vi "ArrayToNum.vi"(6 "输入数组":u8[](array[numeric]) format="%02x", 7 "输入字符串":string) -> (0 "8B":u64, 1 "4B":u32, 2 "2B":u16, 3 "1B":u8)   [LabVIEW 2018]
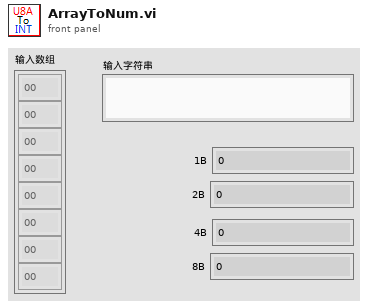
[diagram p1: front panel]
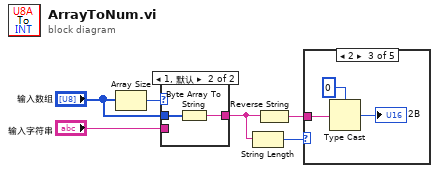
[diagram p0: block diagram]
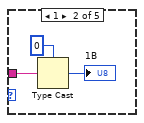
[diagram p4: hidden frame]
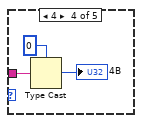
[diagram p5: hidden frame]
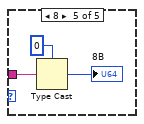
[diagram p6: hidden frame]
diagram:
  n1 = Array Size(array="输入数组") -> (size(s)=w4:i32)
  n2 = case shown="1, 默认" w4 {
    tunnel: "输入数组" -> [_ w9]
    tunnel: [w7 w8] -> w2
    tunnel: "输入字符串" -> [w7 _]
    frame 0 {
    }
    frame 1, Default {
      n3 = Byte Array To String(unsigned byte array=w9) -> (string=w8:string)
    }
  }
  n4 = String Length(string=w2) -> (length=w6:i32)
  n5 = Reverse String(1:w2) -> (0:w5:string)
  n6 = case shown="2" w6 {
    tunnel: w5 -> [_ w12 w15 w18 w19]
    frame 0, Default {
    }
    frame 1 {
      n7 = Type Cast(type=u8 0, x=w12) -> (*(type *) &x=→"1B":u8)
    }
    frame 2 {
      n8 = Type Cast(type=u16 0, x=w15) -> (*(type *) &x=→"2B":u16)
    }
    frame 4 {
      n9 = Type Cast(type=u32 0, x=w18) -> (*(type *) &x=→"4B":u32)
    }
    frame 8 {
      n10 = Type Cast(type=u64 0, x=w19) -> (*(type *) &x=→"8B":u64)
    }
  }
